vi "Calculo_Velocidad.vi"(2 "Tiempo de paso (s)":dbl, 3 "Ejes":i32, 4 "Puntos iniciales de las ventanas":dbl[](array[numeric])) -> (0 "V (m/s)":dbl, 1 "Longitud de la unidad":dbl)   [LabVIEW 2015]
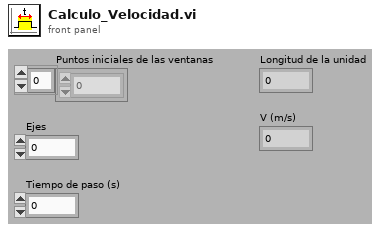
[diagram p1: front panel]
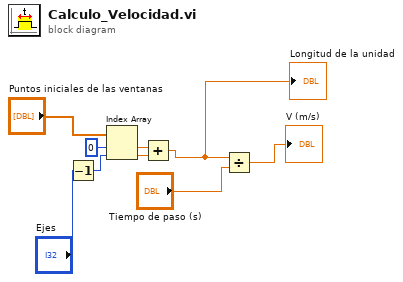
[diagram p0: block diagram]
diagram:
  n1 = Decrement(x="Ejes") -> (x-1=w7:i32)
  n2 = Index Array(array="Puntos iniciales de las ventanas", index #1=0 ("index"), index #2=w7) -> (element #1=w4:dbl, element #2=w3:dbl)
  n3 = Add(x=w4, y=w3) -> (x+y=w5:dbl)
  "Longitud de la unidad" <- w5
  n4 = Divide(x=w5, y="Tiempo de paso (s)") -> (x/y=→"V (m/s)":dbl)
